vi "Arc.vi"(0 "Type":u8(slide)=1 min=1 max=12 step=1 scale=1.0..12.0, 1 "Laser GPIB":u8=10 max=100, 2 "Radius":i32, 3 "Current (mA)":dbl, 4 "Motor GPIB":u8=6, 5 "off delay":u32, 6 "on delay":u32=50) -> ()   [LabVIEW 2010]
uses:
  X-Y Go(Global).vi
panel:
  out "Dummy":string
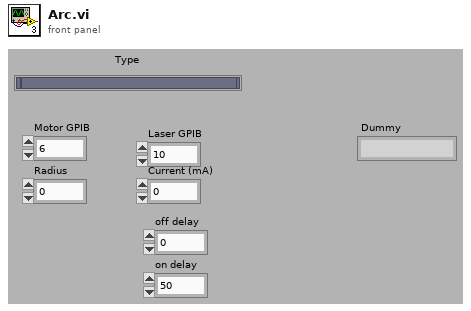
[diagram p1: front panel]
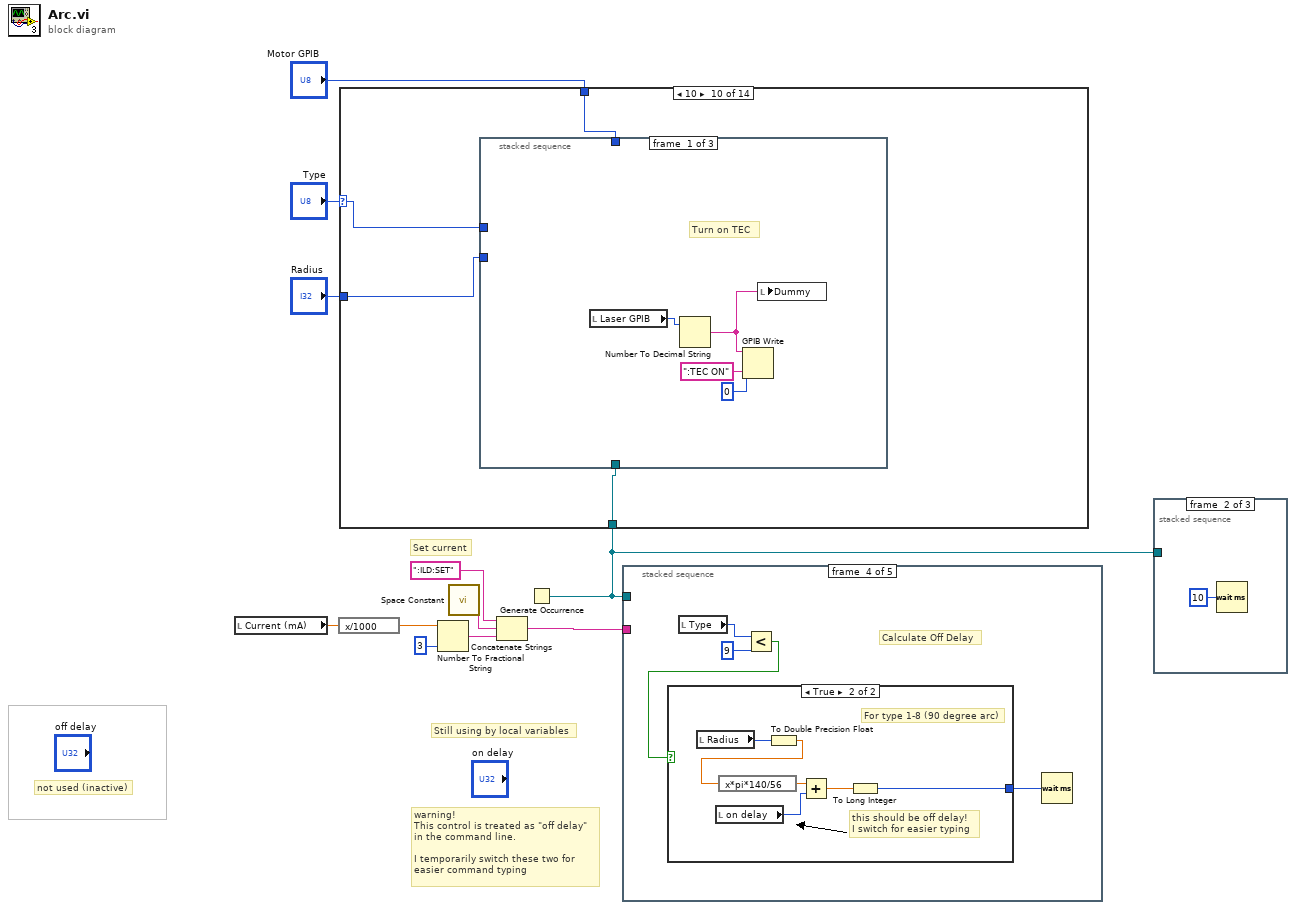
[diagram p0: block diagram]
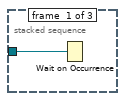
[diagram p2: hidden frame]
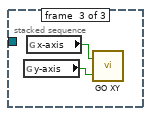
[diagram p3: hidden frame]
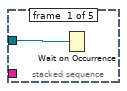
[diagram p4: hidden frame]
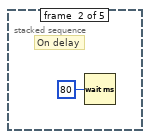
[diagram p5: hidden frame]
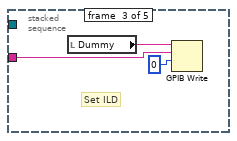
[diagram p6: hidden frame]
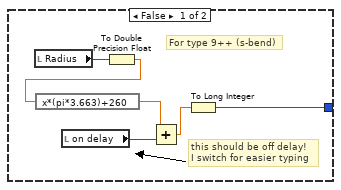
[diagram p7: hidden frame]
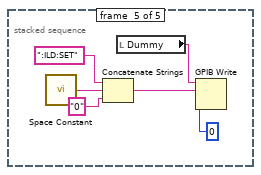
[diagram p8: hidden frame]
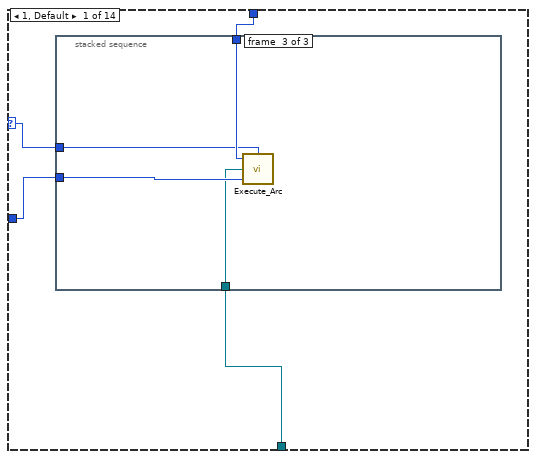
[diagram p9: hidden frame]
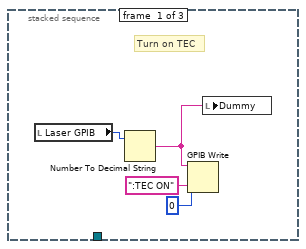
[diagram p10: hidden frame]
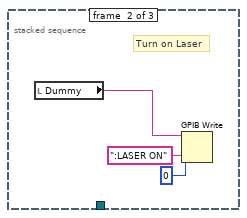
[diagram p11: hidden frame]
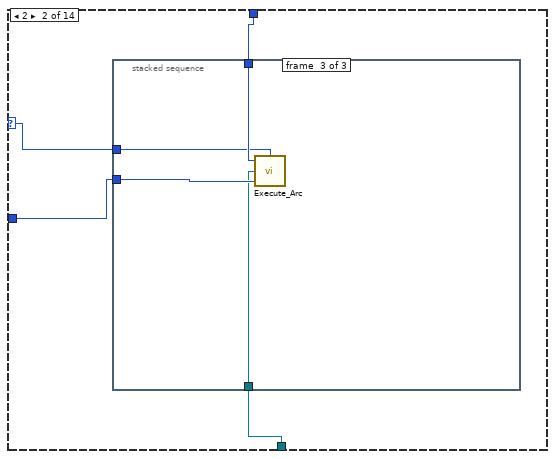
[diagram p12: hidden frame]
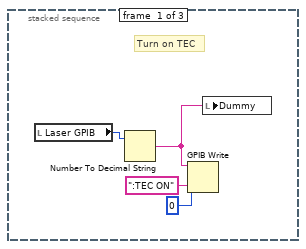
[diagram p13: hidden frame]
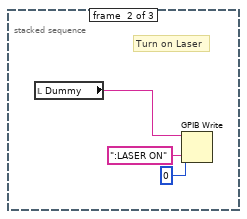
[diagram p14: hidden frame]
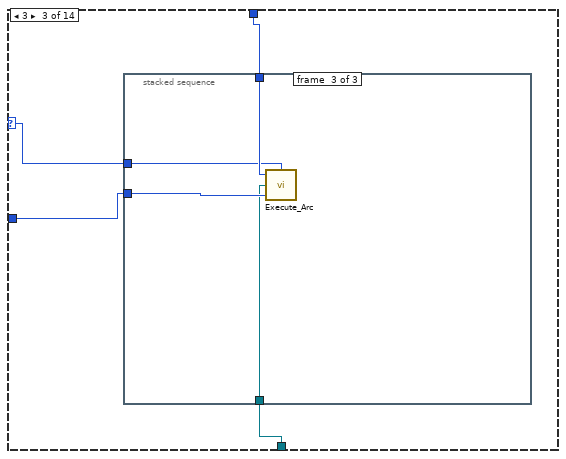
[diagram p15: hidden frame]
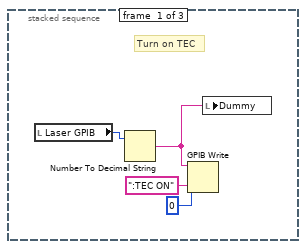
[diagram p16: hidden frame]
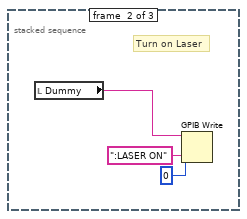
[diagram p17: hidden frame]
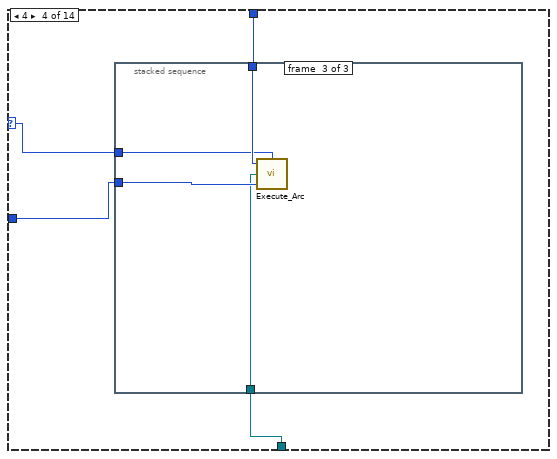
[diagram p18: hidden frame]
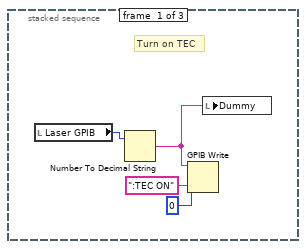
[diagram p19: hidden frame]
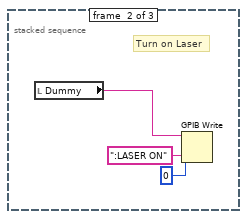
[diagram p20: hidden frame]
diagram:
  # "warning! \nThis control is treated as \"off delay\" \nin the command line.\n\nI temporarily switch these two for\neasier command typing"
  # "not used (inactive)"
  # "Still using by local variables"
  # "Set current"
  n1 = local read "Current (mA)"() -> (w8:dbl)
  n2 = expression code="x/1000"(w8) -> (w5:dbl)
  n3 = Number To Fractional String(number=w5, precision (6)=i16 3) -> (F-format string=w7:string)  [unwired: 2 in]
  n4 = call <vilib>:"Space Constant.vi"() -> ("String"=w3:string)
  n5 = Concatenate Strings(":ILD:SET", w3, w7) -> (w4:string)
  n6 = Generate Occurrence() -> (w1:refnum<k4>)
  n7 = case shown="10" "Type" {
    selector: "Type" -> [w13 w29 w44 w60 w74 w89 w104 w119 w134 w150 w165 w179 _ _]
    tunnel: "Motor GPIB" -> [w15 w30 w45 w58 w75 w90 w105 w120 w135 w147 w163 w180 w193 w226]
    tunnel: "Radius" -> [w14 w28 w43 w59 w73 w88 w103 w118 w133 w149 w164 w178 w192 w225]
    tunnel: w1 -> [w12 w27 w42 w57 w72 w87 w102 w117 w132 w148 w162 w177 _ _]
    frame 1, Default {
      n8 = stacked-sequence {
        tunnel: w15 -> [_ _ w26]
        tunnel: w14 -> [_ _ w25]
        tunnel: w13 -> [_ _ w24]
        tunnel: w12 -> [_ _ w23]
        frame #0 {
          # "Turn on TEC"
          n9 = local read "Laser GPIB"() -> (w17:u8)
          n10 = Number To Decimal String(number=w17) -> (decimal integer string=w16:string)  [unwired: 1 in]
          n11 = GPIB Write(0:w16, 1:":TEC ON" ("data"), 2:i16 0 ("mode (0)")) -> ()  [unwired: 2 in, 2 out]
          n12 = local write "Dummy"(w16) -> ()
        }
        frame #1 {
          # "Turn on Laser"
          n13 = local read "Dummy"() -> (w20:string)
          n14 = GPIB Write(0:w20, 1:":LASER ON" ("data"), 2:i16 0 ("mode (0)")) -> ()  [unwired: 2 in, 2 out]
        }
        frame #2 {
          n15 = call "Execute_Arc.vi"("Type"=w24, "Radius"=w25, "occurrence"=w23, "Motor GPIB"=w26) -> ()  [unwired: 2 in]
        }
      }
    }
    frame 2 {
      n16 = stacked-sequence {
        tunnel: w30 -> [_ _ w41]
        tunnel: w28 -> [_ _ w40]
        tunnel: w29 -> [_ _ w39]
        tunnel: w27 -> [_ _ w38]
        frame #0 {
          # "Turn on TEC"
          n17 = local read "Laser GPIB"() -> (w32:u8)
          n18 = Number To Decimal String(number=w32) -> (decimal integer string=w31:string)  [unwired: 1 in]
          n19 = GPIB Write(0:w31, 1:":TEC ON" ("data"), 2:i16 0 ("mode (0)")) -> ()  [unwired: 2 in, 2 out]
          n20 = local write "Dummy"(w31) -> ()
        }
        frame #1 {
          # "Turn on Laser"
          n21 = local read "Dummy"() -> (w35:string)
          n22 = GPIB Write(0:w35, 1:":LASER ON" ("data"), 2:i16 0 ("mode (0)")) -> ()  [unwired: 2 in, 2 out]
        }
        frame #2 {
          n23 = call "Execute_Arc.vi"("Type"=w39, "Radius"=w40, "occurrence"=w38, "Motor GPIB"=w41) -> ()  [unwired: 2 in]
        }
      }
    }
    frame 3 {
      n24 = stacked-sequence {
        tunnel: w45 -> [_ _ w56]
        tunnel: w43 -> [_ _ w55]
        tunnel: w44 -> [_ _ w54]
        tunnel: w42 -> [_ _ w53]
        frame #0 {
          # "Turn on TEC"
          n25 = local read "Laser GPIB"() -> (w47:u8)
          n26 = Number To Decimal String(number=w47) -> (decimal integer string=w46:string)  [unwired: 1 in]
          n27 = GPIB Write(0:w46, 1:":TEC ON" ("data"), 2:i16 0 ("mode (0)")) -> ()  [unwired: 2 in, 2 out]
          n28 = local write "Dummy"(w46) -> ()
        }
        frame #1 {
          # "Turn on Laser"
          n29 = local read "Dummy"() -> (w50:string)
          n30 = GPIB Write(0:w50, 1:":LASER ON" ("data"), 2:i16 0 ("mode (0)")) -> ()  [unwired: 2 in, 2 out]
        }
        frame #2 {
          n31 = call "Execute_Arc.vi"("Type"=w54, "Radius"=w55, "occurrence"=w53, "Motor GPIB"=w56) -> ()  [unwired: 2 in]
        }
      }
    }
    frame 4 {
      n32 = stacked-sequence {
        tunnel: w58 -> [_ _ w71]
        tunnel: w59 -> [_ _ w70]
        tunnel: w60 -> [_ _ w69]
        tunnel: w57 -> [_ _ w68]
        frame #0 {
          # "Turn on TEC"
          n33 = local read "Laser GPIB"() -> (w62:u8)
          n34 = Number To Decimal String(number=w62) -> (decimal integer string=w61:string)  [unwired: 1 in]
          n35 = GPIB Write(0:w61, 1:":TEC ON" ("data"), 2:i16 0 ("mode (0)")) -> ()  [unwired: 2 in, 2 out]
          n36 = local write "Dummy"(w61) -> ()
        }
        frame #1 {
          # "Turn on Laser"
          n37 = local read "Dummy"() -> (w65:string)
          n38 = GPIB Write(0:w65, 1:":LASER ON" ("data"), 2:i16 0 ("mode (0)")) -> ()  [unwired: 2 in, 2 out]
        }
        frame #2 {
          n39 = call "Execute_Arc.vi"("Type"=w69, "Radius"=w70, "occurrence"=w68, "Motor GPIB"=w71) -> ()  [unwired: 2 in]
        }
      }
    }
    frame 5 {
      n40 = stacked-sequence {
        tunnel: w75 -> [_ _ w86]
        tunnel: w73 -> [_ _ w85]
        tunnel: w74 -> [_ _ w84]
        tunnel: w72 -> [_ _ w83]
        frame #0 {
          # "Turn on TEC"
          n41 = local read "Laser GPIB"() -> (w77:u8)
          n42 = Number To Decimal String(number=w77) -> (decimal integer string=w76:string)  [unwired: 1 in]
          n43 = GPIB Write(0:w76, 1:":TEC ON" ("data"), 2:i16 0 ("mode (0)")) -> ()  [unwired: 2 in, 2 out]
          n44 = local write "Dummy"(w76) -> ()
        }
        frame #1 {
          # "Turn on Laser"
          n45 = local read "Dummy"() -> (w80:string)
          n46 = GPIB Write(0:w80, 1:":LASER ON" ("data"), 2:i16 0 ("mode (0)")) -> ()  [unwired: 2 in, 2 out]
        }
        frame #2 {
          n47 = call "Execute_Arc.vi"("Type"=w84, "Radius"=w85, "occurrence"=w83, "Motor GPIB"=w86) -> ()  [unwired: 2 in]
        }
      }
    }
    frame 6 {
      n48 = stacked-sequence {
        tunnel: w90 -> [_ _ w101]
        tunnel: w88 -> [_ _ w100]
        tunnel: w89 -> [_ _ w99]
        tunnel: w87 -> [_ _ w98]
        frame #0 {
          # "Turn on TEC"
          n49 = local read "Laser GPIB"() -> (w92:u8)
          n50 = Number To Decimal String(number=w92) -> (decimal integer string=w91:string)  [unwired: 1 in]
          n51 = GPIB Write(0:w91, 1:":TEC ON" ("data"), 2:i16 0 ("mode (0)")) -> ()  [unwired: 2 in, 2 out]
          n52 = local write "Dummy"(w91) -> ()
        }
        frame #1 {
          # "Turn on Laser"
          n53 = local read "Dummy"() -> (w95:string)
          n54 = GPIB Write(0:w95, 1:":LASER ON" ("data"), 2:i16 0 ("mode (0)")) -> ()  [unwired: 2 in, 2 out]
        }
        frame #2 {
          n55 = call "Execute_Arc.vi"("Type"=w99, "Radius"=w100, "occurrence"=w98, "Motor GPIB"=w101) -> ()  [unwired: 2 in]
        }
      }
    }
    frame 7 {
      n56 = stacked-sequence {
        tunnel: w105 -> [_ _ w116]
        tunnel: w103 -> [_ _ w115]
        tunnel: w104 -> [_ _ w114]
        tunnel: w102 -> [_ _ w113]
        frame #0 {
          # "Turn on TEC"
          n57 = local read "Laser GPIB"() -> (w107:u8)
          n58 = Number To Decimal String(number=w107) -> (decimal integer string=w106:string)  [unwired: 1 in]
          n59 = GPIB Write(0:w106, 1:":TEC ON" ("data"), 2:i16 0 ("mode (0)")) -> ()  [unwired: 2 in, 2 out]
          n60 = local write "Dummy"(w106) -> ()
        }
        frame #1 {
          # "Turn on Laser"
          n61 = local read "Dummy"() -> (w110:string)
          n62 = GPIB Write(0:w110, 1:":LASER ON" ("data"), 2:i16 0 ("mode (0)")) -> ()  [unwired: 2 in, 2 out]
        }
        frame #2 {
          n63 = call "Execute_Arc.vi"("Type"=w114, "Radius"=w115, "occurrence"=w113, "Motor GPIB"=w116) -> ()  [unwired: 2 in]
        }
      }
    }
    frame 8 {
      n64 = stacked-sequence {
        tunnel: w120 -> [_ _ w131]
        tunnel: w118 -> [_ _ w130]
        tunnel: w119 -> [_ _ w129]
        tunnel: w117 -> [_ _ w128]
        frame #0 {
          # "Turn on TEC"
          n65 = local read "Laser GPIB"() -> (w122:u8)
          n66 = Number To Decimal String(number=w122) -> (decimal integer string=w121:string)  [unwired: 1 in]
          n67 = GPIB Write(0:w121, 1:":TEC ON" ("data"), 2:i16 0 ("mode (0)")) -> ()  [unwired: 2 in, 2 out]
          n68 = local write "Dummy"(w121) -> ()
        }
        frame #1 {
          # "Turn on Laser"
          n69 = local read "Dummy"() -> (w125:string)
          n70 = GPIB Write(0:w125, 1:":LASER ON" ("data"), 2:i16 0 ("mode (0)")) -> ()  [unwired: 2 in, 2 out]
        }
        frame #2 {
          n71 = call "Execute_Arc.vi"("Type"=w129, "Radius"=w130, "occurrence"=w128, "Motor GPIB"=w131) -> ()  [unwired: 2 in]
        }
      }
    }
    frame 9 {
      n72 = stacked-sequence {
        tunnel: w135 -> [_ _ w146]
        tunnel: w133 -> [_ _ w145]
        tunnel: w134 -> [_ _ w144]
        tunnel: w132 -> [_ _ w143]
        frame #0 {
          # "Turn on TEC"
          n73 = local read "Laser GPIB"() -> (w137:u8)
          n74 = Number To Decimal String(number=w137) -> (decimal integer string=w136:string)  [unwired: 1 in]
          n75 = GPIB Write(0:w136, 1:":TEC ON" ("data"), 2:i16 0 ("mode (0)")) -> ()  [unwired: 2 in, 2 out]
          n76 = local write "Dummy"(w136) -> ()
        }
        frame #1 {
          # "Turn on Laser"
          n77 = local read "Dummy"() -> (w140:string)
          n78 = GPIB Write(0:w140, 1:":LASER ON" ("data"), 2:i16 0 ("mode (0)")) -> ()  [unwired: 2 in, 2 out]
        }
        frame #2 {
          n79 = call "Execute_Arc.vi"("Type"=w144, "Radius"=w145, "occurrence"=w143, "Motor GPIB"=w146) -> ()  [unwired: 2 in]
        }
      }
    }
    frame 10 {
      n80 = stacked-sequence {
        tunnel: w147 -> [_ _ w161]
        tunnel: w149 -> [_ _ w160]
        tunnel: w150 -> [_ _ w159]
        tunnel: w148 -> [_ _ w158]
        frame #0 {
          # "Turn on TEC"
          n81 = local read "Laser GPIB"() -> (w152:u8)
          n82 = Number To Decimal String(number=w152) -> (decimal integer string=w151:string)  [unwired: 1 in]
          n83 = GPIB Write(0:w151, 1:":TEC ON" ("data"), 2:i16 0 ("mode (0)")) -> ()  [unwired: 2 in, 2 out]
          n84 = local write "Dummy"(w151) -> ()
        }
        frame #1 {
          # "Turn on Laser"
          n85 = local read "Dummy"() -> (w155:string)
          n86 = GPIB Write(0:w155, 1:":LASER ON" ("data"), 2:i16 0 ("mode (0)")) -> ()  [unwired: 2 in, 2 out]
        }
        frame #2 {
          n87 = call "Execute_Arc.vi"("Type"=w159, "Radius"=w160, "occurrence"=w158, "Motor GPIB"=w161) -> ()  [unwired: 2 in]
        }
      }
    }
    frame 11 {
      n88 = stacked-sequence {
        tunnel: w163 -> [_ _ w176]
        tunnel: w164 -> [_ _ w175]
        tunnel: w165 -> [_ _ w174]
        tunnel: w162 -> [_ _ w173]
        frame #0 {
          # "Turn on TEC"
          n89 = local read "Laser GPIB"() -> (w167:u8)
          n90 = Number To Decimal String(number=w167) -> (decimal integer string=w166:string)  [unwired: 1 in]
          n91 = GPIB Write(0:w166, 1:":TEC ON" ("data"), 2:i16 0 ("mode (0)")) -> ()  [unwired: 2 in, 2 out]
          n92 = local write "Dummy"(w166) -> ()
        }
        frame #1 {
          # "Turn on Laser"
          n93 = local read "Dummy"() -> (w170:string)
          n94 = GPIB Write(0:w170, 1:":LASER ON" ("data"), 2:i16 0 ("mode (0)")) -> ()  [unwired: 2 in, 2 out]
        }
        frame #2 {
          n95 = call "Execute_Arc.vi"("Type"=w174, "Radius"=w175, "occurrence"=w173, "Motor GPIB"=w176) -> ()  [unwired: 2 in]
        }
      }
    }
    frame 12 {
      n96 = stacked-sequence {
        tunnel: w180 -> [_ _ w191]
        tunnel: w178 -> [_ _ w190]
        tunnel: w179 -> [_ _ w189]
        tunnel: w177 -> [_ _ w188]
        frame #0 {
          # "Turn on TEC"
          n97 = local read "Laser GPIB"() -> (w182:u8)
          n98 = Number To Decimal String(number=w182) -> (decimal integer string=w181:string)  [unwired: 1 in]
          n99 = GPIB Write(0:w181, 1:":TEC ON" ("data"), 2:i16 0 ("mode (0)")) -> ()  [unwired: 2 in, 2 out]
          n100 = local write "Dummy"(w181) -> ()
        }
        frame #1 {
          # "Turn on Laser"
          n101 = local read "Dummy"() -> (w185:string)
          n102 = GPIB Write(0:w185, 1:":LASER ON" ("data"), 2:i16 0 ("mode (0)")) -> ()  [unwired: 2 in, 2 out]
        }
        frame #2 {
          n103 = call "Execute_Arc.vi"("Type"=w189, "Radius"=w190, "occurrence"=w188, "Motor GPIB"=w191) -> ()  [unwired: 2 in]
        }
      }
    }
    frame 13 {
      n104 = disable-structure shown="Disabled" {
        disable-tunnel: w193 -> [w195 _]
        disable-tunnel: w192 -> [w194 _]
        frame Disabled {
          # "Full circle anticlockwise"
          n105 = stacked-sequence {
            tunnel: w195 -> [_ _ _ w213 _]
            tunnel: w194 -> [_ _ _ w212 _]
            frame #0 {
              # "Turn on TEC"
              n106 = Number To Decimal String(number="Laser GPIB") -> (decimal integer string=w196:string)  [unwired: 1 in]
              "Dummy" <- w196
              n107 = GPIB Write(0:w196, 1:":TEC ON" ("data"), 2:i16 0 ("mode (0)")) -> ()  [unwired: 2 in, 2 out]
            }
            frame #1 {
              # "Turn on Laser"
              n108 = local read "Dummy"() -> (w200:string)
              n109 = GPIB Write(0:w200, 1:":LASER ON" ("data"), 2:i16 0 ("mode (0)")) -> ()  [unwired: 2 in, 2 out]
            }
            frame #2 {
              # "Set current"
              n110 = expression code="x/1000"("Current (mA)") -> (w207:dbl)
              n111 = call <vilib>:"Space Constant.vi"() -> ("String"=w209:string)
              n112 = Number To Fractional String(number=w207, precision (6)=i16 3) -> (F-format string=w204:string)  [unwired: 2 in]
              n113 = Concatenate Strings(":ILD:SET", w209, w204) -> (w208:string)
              n114 = local read "Dummy"() -> (w203:string)
              n115 = GPIB Write(0:w203, 1:w208, 2:i16 0 ("mode (0)")) -> ()  [unwired: 2 in, 2 out]
            }
            frame #3 {
              n116 = for {
                N: 4 -> [_]
                tunnel: w213 -> [w216]
                tunnel: w212 -> [w215]
                i -> [w218]
                n117 = Increment(x=w218) -> (x+1=w217:i32)
                n118 = call "Execute_Arc.vi"("Type"=w217, "Radius"=w215, "Motor GPIB"=w216) -> ()  [unwired: 1 in]
              }
            }
            frame #4 {
              # "Set current to 0"
              n119 = call <vilib>:"Space Constant.vi"() -> ("String"=w222:string)
              n120 = Concatenate Strings(":ILD:SET", w222, "0" ("string")) -> (w221:string)
              n121 = local read "Dummy"() -> (w220:string)
              n122 = GPIB Write(0:w220, 1:w221, 2:i16 0 ("mode (0)")) -> ()  [unwired: 2 in, 2 out]
            }
          }
        }
        frame Enabled {
        }
      }
    }
    frame 14 {
      n123 = disable-structure shown="Disabled" {
        disable-tunnel: w226 -> [w228 _]
        disable-tunnel: w225 -> [w227 _]
        frame Disabled {
          n124 = stacked-sequence {
            tunnel: w228 -> [_ _ _ w246 _]
            tunnel: w227 -> [_ _ _ w245 _]
            frame #0 {
              # "Turn on TEC"
              n125 = local read "Laser GPIB"() -> (w230:u8)
              n126 = Number To Decimal String(number=w230) -> (decimal integer string=w229:string)  [unwired: 1 in]
              n127 = GPIB Write(0:w229, 1:":TEC ON" ("data"), 2:i16 0 ("mode (0)")) -> ()  [unwired: 2 in, 2 out]
              n128 = local write "Dummy"(w229) -> ()
            }
            frame #1 {
              # "Turn on Laser"
              n129 = local read "Dummy"() -> (w233:string)
              n130 = GPIB Write(0:w233, 1:":LASER ON" ("data"), 2:i16 0 ("mode (0)")) -> ()  [unwired: 2 in, 2 out]
            }
            frame #2 {
              # "Set current"
              n131 = local read "Current (mA)"() -> (w236:dbl)
              n132 = expression code="x/1000"(w236) -> (w240:dbl)
              n133 = call <vilib>:"Space Constant.vi"() -> ("String"=w242:string)
              n134 = Number To Fractional String(number=w240, precision (6)=i16 3) -> (F-format string=w238:string)  [unwired: 2 in]
              n135 = Concatenate Strings(":ILD:SET", w242, w238) -> (w241:string)
              n136 = local read "Dummy"() -> (w237:string)
              n137 = GPIB Write(0:w237, 1:w241, 2:i16 0 ("mode (0)")) -> ()  [unwired: 2 in, 2 out]
            }
            frame #3 {
              n138 = for {
                N: 4 -> [_]
                tunnel: w246 -> [w251]
                tunnel: w245 -> [w250]
                i -> [w249]
                n139 = expression code="x+5"(w249) -> (w248:i32)
                n140 = call "Execute_Arc.vi"("Type"=w248, "Radius"=w250, "Motor GPIB"=w251) -> ()  [unwired: 1 in]
              }
            }
            frame #4 {
              # "Set current to 0"
              n141 = call <vilib>:"Space Constant.vi"() -> ("String"=w255:string)
              n142 = Concatenate Strings(":ILD:SET", w255, "0" ("string")) -> (w254:string)
              n143 = local read "Dummy"() -> (w253:string)
              n144 = GPIB Write(0:w253, 1:w254, 2:i16 0 ("mode (0)")) -> ()  [unwired: 2 in, 2 out]
            }
          }
        }
        frame Enabled {
        }
      }
    }
  }
  n145 = stacked-sequence {
    tunnel: w4 -> [_ _ w261 _ _]
    tunnel: w1 -> [w258 _ _ _ _]
    frame #0 {
      n146 = Wait on Occurrence(2:w258) -> ()  [unwired: 2 in, 1 out]
    }
    frame #1 {
      # "On delay"
      n147 = Wait (ms)(milliseconds to wait=u32 80) -> ()  [unwired: 1 out]
    }
    frame #2 {
      # "Set ILD"
      n148 = local read "Dummy"() -> (w262:string)
      n149 = GPIB Write(0:w262, 1:w261, 2:i16 0 ("mode (0)")) -> ()  [unwired: 2 in, 2 out]
    }
    frame #3 {
      # "Calculate Off Delay"
      n150 = local read "Type"() -> (w263:u8)
      n151 = Less?(x=w263, y=u8 9) -> (x < y?=w265:bool)
      n152 = case shown="True" w265 {
        tunnel: [w267 w273] -> w264
        frame False {
          # "this should be off delay!\nI switch for easier typing"
          # "For type 9++ (s-bend)"
          n153 = local read "Radius"() -> (w272:i32)
          n154 = local read "on delay"() -> (w269:u32)
          n155 = To Double Precision Float(number=w272) -> (double precision float=w271:dbl)
          n156 = expression code="x*(pi*3.663)+260"(w271) -> (w270:dbl)
          n157 = Add(x=w270, y=w269) -> (x+y=w268:dbl)
          n158 = To Long Integer(number=w268) -> (32bit integer=w267:i32)
        }
        frame True {
          # "this should be off delay!\nI switch for easier typing"
          # "For type 1-8 (90 degree arc)"
          n159 = local read "Radius"() -> (w278:i32)
          n160 = local read "on delay"() -> (w275:u32)
          n161 = To Double Precision Float(number=w278) -> (double precision float=w277:dbl)
          n162 = expression code="x*pi*140/56"(w277) -> (w276:dbl)
          n163 = Add(x=w276, y=w275) -> (x+y=w274:dbl)
          n164 = To Long Integer(number=w274) -> (32bit integer=w273:i32)
        }
      }
      n165 = Wait (ms)(milliseconds to wait=w264) -> ()  [unwired: 1 out]
    }
    frame #4 {
      n166 = call <vilib>:"Space Constant.vi"() -> ("String"=w281:string)
      n167 = Concatenate Strings(":ILD:SET", w281, "0" ("string")) -> (w282:string)
      n168 = local read "Dummy"() -> (w283:string)
      n169 = GPIB Write(0:w283, 1:w282, 2:i16 0 ("mode (0)")) -> ()  [unwired: 2 in, 2 out]
    }
  }
  n170 = stacked-sequence {
    tunnel: w1 -> [w285 _ _]
    frame #0 {
      n171 = Wait on Occurrence(2:w285) -> ()  [unwired: 2 in, 1 out]
    }
    frame #1 {
      n172 = Wait (ms)(milliseconds to wait=u32 10) -> ()  [unwired: 1 out]
    }
    frame #2 {
      n173 = global read "X-Y Go(Global).vi" "y-axis"() -> (w287:bool)
      n174 = global read "X-Y Go(Global).vi" "x-axis"() -> (w288:bool)
      n175 = call "GO XY.vi"("Y-axis"=w287, "X-axis"=w288) -> ()  [unwired: 1 in]
    }
  }
